vi "maintenancePIP.vi"(8 "error in (no error)":errorcluster) -> (0 "error out":errorcluster, 3 "MAINTENANCE MODE-8, 9, 10, 11":string)   [LabVIEW 2018]
uses:
  Global_1259.vi
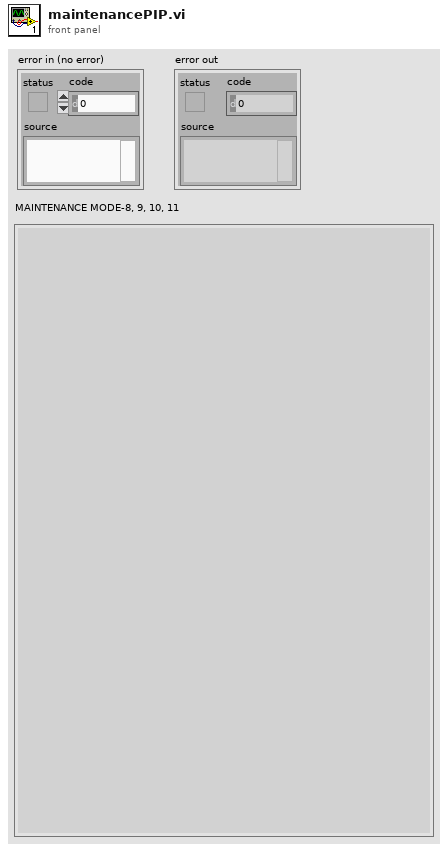
[diagram p1: front panel]
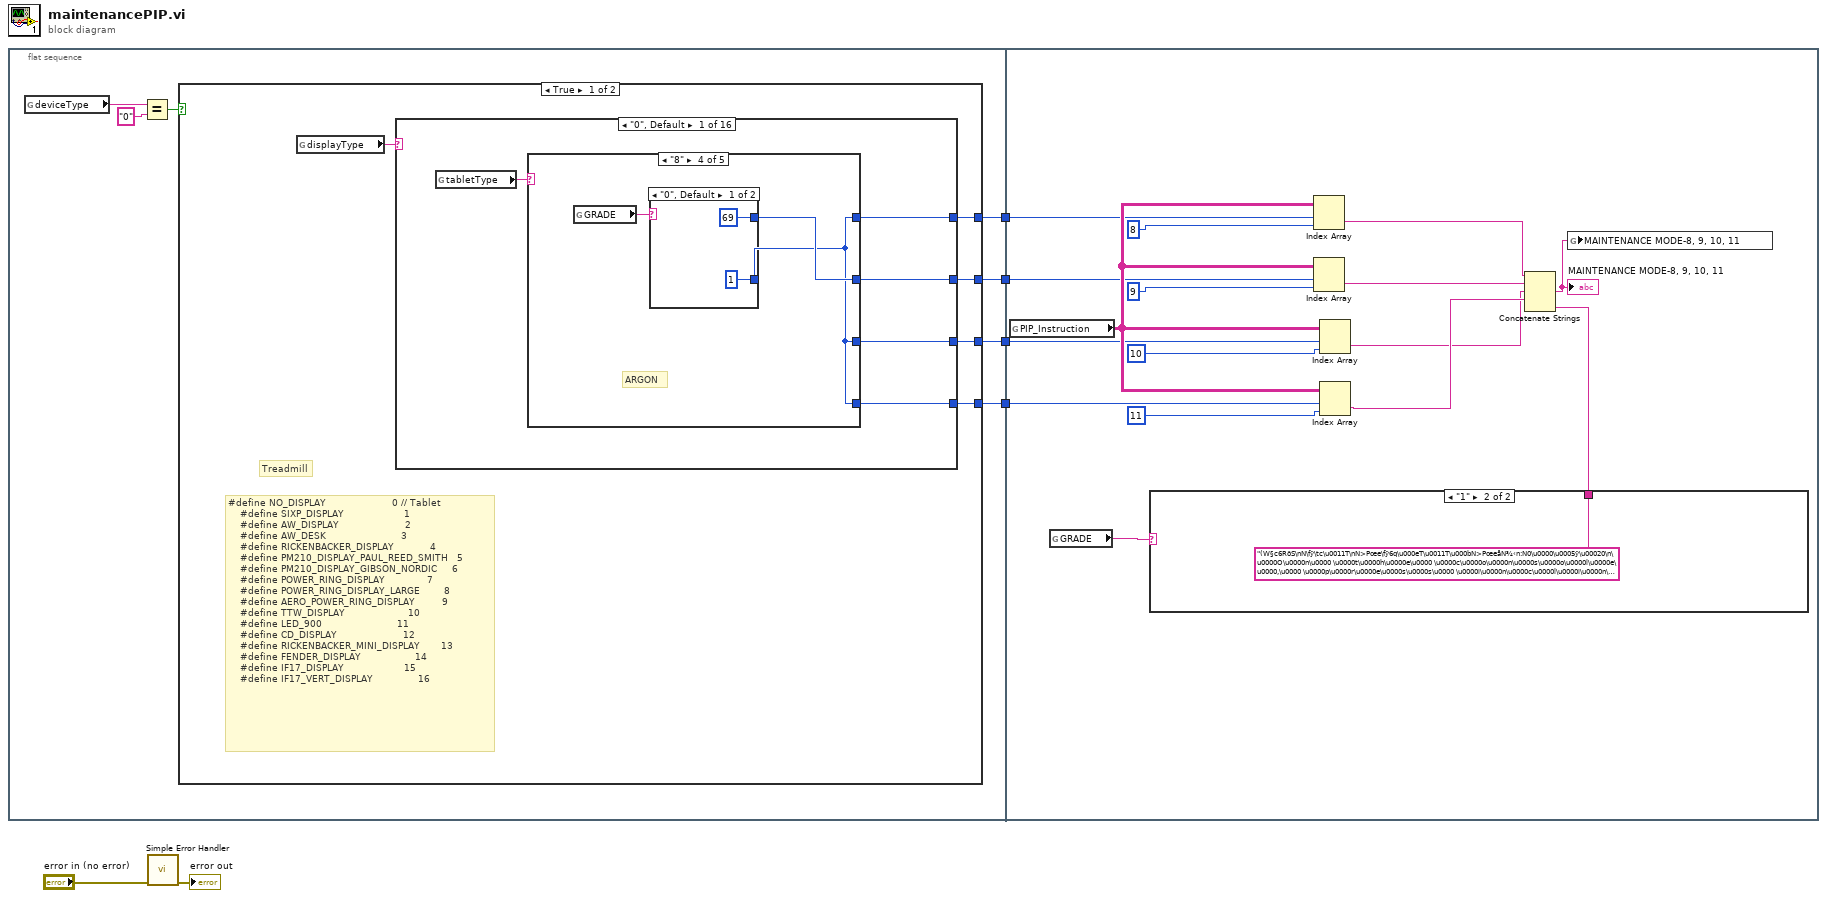
[diagram p0: block diagram]
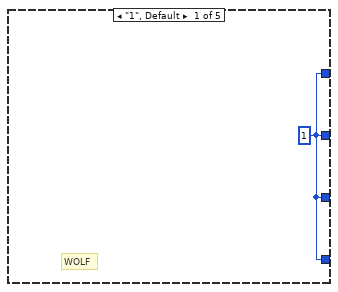
[diagram p2: hidden frame]
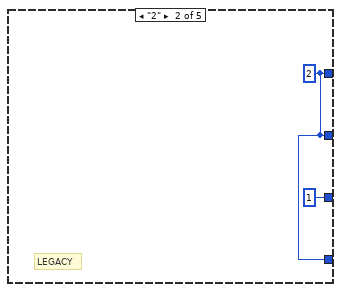
[diagram p3: hidden frame]
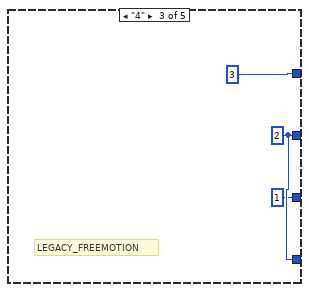
[diagram p4: hidden frame]
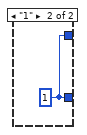
[diagram p5: hidden frame]
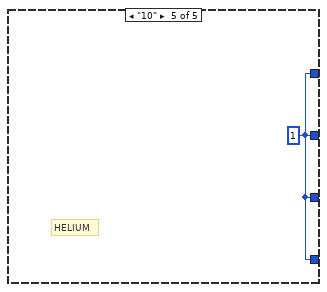
[diagram p6: hidden frame]
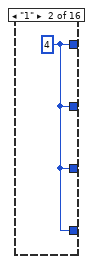
[diagram p7: hidden frame]
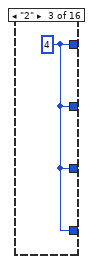
[diagram p8: hidden frame]
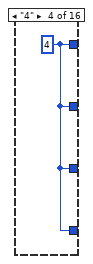
[diagram p9: hidden frame]
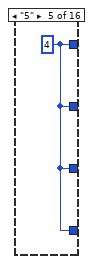
[diagram p10: hidden frame]
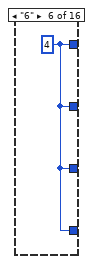
[diagram p11: hidden frame]
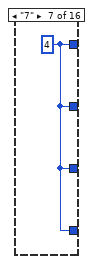
[diagram p12: hidden frame]
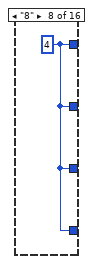
[diagram p13: hidden frame]
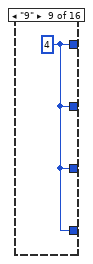
[diagram p14: hidden frame]
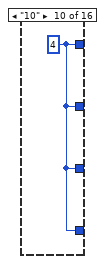
[diagram p15: hidden frame]
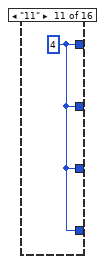
[diagram p16: hidden frame]
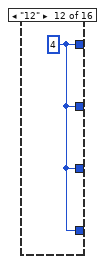
[diagram p17: hidden frame]
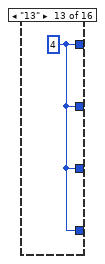
[diagram p18: hidden frame]
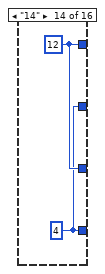
[diagram p19: hidden frame]
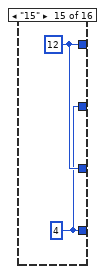
[diagram p20: hidden frame]
diagram:
  n1 = flat-sequence {
    tunnel: [w13] -> w6
    tunnel: [w12] -> w5
    tunnel: [w11] -> w4
    tunnel: [w10] -> w3
    tunnel: w6 -> [w155]
    tunnel: w5 -> [w154]
    tunnel: w4 -> [w153]
    tunnel: w3 -> [w152]
    frame #0 {
      n2 = global read "Global_1259.vi" "deviceType"() -> (w9:string)
      n3 = Equal?(x=w9, y="0") -> (x = y?=w7:bool)
      n4 = case shown="True" w7 {
        tunnel: [w18 w58] -> w13
        tunnel: [w17 w57] -> w12
        tunnel: [w16 w56] -> w11
        tunnel: [w15 w55] -> w10
        frame True {
          # "#define NO_DISPLAY                      0 // Tablet\n    #define SIXP_DISPLAY                    1\n    #define AW_DISPLAY                      2\n    #define AW_DESK                         3\n    #define RICKENBACKER_DISPLAY            4\n    #define PM210_DISPLAY_PAUL_REED_SMITH   5\n    #define PM210_DISPLAY_GIBSON_NORDIC     6\n    #define POWER_RING_DISPLAY              7\n    #define POWER_RING_DISPLAY_LARGE        8\n    #define AERO_POWER_RING_DISPLAY         9\n    #define TTW_DISPLAY                     10\n    #define LED_900                         11\n    #define CD_DISPLAY                      12\n    #define RICKENBACKER_MINI_DISPLAY       13\n    #define FENDER_DISPLAY                  14\n    #define IF17_DISPLAY                    15\n    #define IF17_VERT_DISPLAY               16"
          # "Treadmill"
          n5 = global read "Global_1259.vi" "displayType"() -> (w14:string)
          n6 = case shown="\"0\", Default" w14 {
            tunnel: [w22 w37 w38 w39 w40 w41 w42 w43 w44 w45 w46 w47 w48 w50 w52 w53] -> w18
            tunnel: [w21 w37 w38 w39 w40 w41 w42 w43 w44 w45 w46 w47 w48 w49 w51 w54] -> w17
            tunnel: [w20 w37 w38 w39 w40 w41 w42 w43 w44 w45 w46 w47 w48 w50 w52 w53] -> w16
            tunnel: [w19 w37 w38 w39 w40 w41 w42 w43 w44 w45 w46 w47 w48 w49 w51 w54] -> w15
            frame "0", Default {
              n7 = global read "Global_1259.vi" "tabletType"() -> (w23:string)
              n8 = case shown="\"8\"" w23 {
                tunnel: [w24 w25 w28 w31 w36] -> w21
                tunnel: [w24 w25 3 w30 w36] -> w22
                tunnel: [w24 1 1 w30 w36] -> w20
                tunnel: [w24 w25 w28 w30 w36] -> w19
                frame "1", Default {
                  w24 = 1
                  # "WOLF"
                }
                frame "2" {
                  w25 = 2
                  # "LEGACY"
                }
                frame "4" {
                  w28 = 2
                  # "LEGACY_FREEMOTION"
                }
                frame "8" {
                  # "ARGON"
                  n9 = global read "Global_1259.vi" "GRADE"() -> (w32:string)
                  n10 = case shown="\"0\", Default" w32 {
                    tunnel: [1 w35] -> w30
                    tunnel: [69 w35] -> w31
                    frame "0", Default {
                    }
                    frame "1" {
                      w35 = 1
                    }
                  }
                }
                frame "10" {
                  w36 = 1
                  # "HELIUM"
                }
              }
            }
            frame "1" {
              w37 = 4
            }
            frame "2" {
              w38 = 4
            }
            frame "4" {
              w39 = 4
            }
            frame "5" {
              w40 = 4
            }
            frame "6" {
              w41 = 4
            }
            frame "7" {
              w42 = 4
            }
            frame "8" {
              w43 = 4
            }
            frame "9" {
              w44 = 4
            }
            frame "10" {
              w45 = 4
            }
            frame "11" {
              w46 = 4
            }
            frame "12" {
              w47 = 4
            }
            frame "13" {
              w48 = 4
            }
            frame "14" {
              w49 = 4
              w50 = 12
            }
            frame "15" {
              w51 = 4
              w52 = 12
            }
            frame "16" {
              w54 = 4
              w53 = 12
            }
          }
        }
        frame False {
          # "not treadmill"
          n11 = global read "Global_1259.vi" "displayType"() -> (w61:string)
          n12 = Equal?(x=w61, y="0") -> (x = y?=w59:bool)
          n13 = case shown="False" w59 {
            tunnel: [w65 w123] -> w58
            tunnel: [w66 w122] -> w57
            tunnel: [w64 w121] -> w56
            tunnel: [w63 w120] -> w55
            frame False {
              n14 = global read "Global_1259.vi" "GRADE"() -> (w62:string)
              n15 = case shown="\"0\", Default" w62 {
                tunnel: [w69 w97] -> w66
                tunnel: [w70 w96] -> w65
                tunnel: [w68 w95] -> w64
                tunnel: [w67 w94] -> w63
                frame "0", Default {
                  n16 = global read "Global_1259.vi" "buttonType"() -> (w71:string)
                  n17 = case shown="\"2\"" w71 {
                    tunnel: [8 7 10 7 7 w92] -> w68
                    tunnel: [7 7 10 7 7 w92] -> w67
                    tunnel: [69 69 69 69 69 w92] -> w69
                    tunnel: [8 7 10 8 7 w92] -> w70
                    frame "1", Default {
                    }
                    frame "2" {
                    }
                    frame "4" {
                    }
                    frame "9" {
                    }
                    frame "10" {
                    }
                    frame "12" {
                      w92 = 69
                    }
                  }
                }
                frame "1" {
                  n18 = global read "Global_1259.vi" "buttonType"() -> (w93:string)
                  n19 = case shown="\"2\"" w93 {
                    tunnel: [8 7 10 7 7 w118] -> w95
                    tunnel: [7 7 10 7 7 w118] -> w94
                    tunnel: [7 7 69 8 7 w118] -> w97
                    tunnel: [8 7 10 8 7 w118] -> w96
                    frame "1", Default {
                    }
                    frame "2" {
                    }
                    frame "4" {
                    }
                    frame "9" {
                    }
                    frame "10" {
                    }
                    frame "12" {
                      w118 = 69
                    }
                  }
                }
              }
            }
            frame True {
              n20 = global read "Global_1259.vi" "TABLET"() -> (w119:string)
              n21 = case shown="\"1\", Default" w119 {
                tunnel: [w131 w133 w138 w139 w145] -> w123
                tunnel: [w131 w132 w138 w140 w145] -> w122
                tunnel: [w131 w132 w138 w139 w145] -> w121
                tunnel: [w131 w132 w138 w139 w145] -> w120
                frame "1", Default {
                  w131 = 1
                  n22 = global read "Global_1259.vi" "PIP_Instruction"() -> (w130:string[][])
                  n23 = Index Array(array=w130, index (row)=1 ("disabled index (row)"), index (col)=16 ("disabled index (col)")) -> (element=w129:string)
                  n24 = Index Array(array=w130, index (row)=1 ("disabled index (row)"), index (col)=20 ("disabled index (col)")) -> (element=w128:string)
                  n25 = global write "Global_1259.vi" "USB-16"(w129) -> ()
                  n26 = global write "Global_1259.vi" "TV-20"(w128) -> ()
                }
                frame "2" {
                  n27 = global read "Global_1259.vi" "GRADE"() -> (w134:string)
                  n28 = case shown="\"0\", Default" w134 {
                    tunnel: [1 w137] -> w133
                    tunnel: [69 w137] -> w132
                    frame "0", Default {
                    }
                    frame "1" {
                      w137 = 1
                    }
                  }
                }
                frame "4" {
                  w138 = 1
                }
                frame "8" {
                  n29 = global read "Global_1259.vi" "GRADE"() -> (w141:string)
                  n30 = case shown="\"0\", Default" w141 {
                    tunnel: [1 w144] -> w139
                    tunnel: [69 w144] -> w140
                    frame "0", Default {
                    }
                    frame "1" {
                      w144 = 1
                    }
                  }
                }
                frame "16" {
                  w145 = 1
                }
              }
            }
          }
        }
      }
    }
    frame #1 {
      n31 = global read "Global_1259.vi" "PIP_Instruction"() -> (w161:string[][])
      n32 = global read "Global_1259.vi" "GRADE"() -> (w146:string)
      n33 = case shown="\"1\"" w146 {
        tunnel: ["None" "(W§c6RðS\nN\fÿ\tc\u0011T\nN>Pœe\fÿ6q\u000eT\u0011T\u000bN>PœeåN¾‹n:N0\u0000\u0005ÿ\u00020\n\u0000O\u0000n\u0000 \u0000t\u0000h\u0000e\u0000 \u0000c\u0000o\u0000n\u0000s\u0000o\u0000l\u0000e\u0000,\u0000 \u0000p\u0000r\u0000e\u0000s\u0000s\u0000 \u0000i\u0000n\u0000c\u0000l\u0000i\u0000n\u0000e\u0000 \u0000u\u0000p\u0000 \u0000a\u0000n\u0000d\u0000 \u0000t\u0000h\u0000e\u0000n\u0000 \u0000i\u0000n\u0000c\u0000l\u0000i\u0000n\u0000e\u0000 \u0000d\u0000o\u0000w\u0000n\u0000 \u0000t\u0000o\u0000 \u0000s\u0000e\u0000t\u0000 \u0000t\u0000o\u0000 \u00000\u0000%\u0000.\u0000"] -> w147
        frame "0", Default {
        }
        frame "1" {
        }
      }
      n34 = Index Array(array=w161, index (row)=w155, index (col)=8 ("disabled index (col)")) -> (element=w151:string)
      n35 = Index Array(array=w161, index (row)=w154, index (col)=9 ("disabled index (col)")) -> (element=w150:string)
      n36 = Index Array(array=w161, index (row)=w153, index (col)=10 ("disabled index (col)")) -> (element=w148:string)
      n37 = Index Array(array=w161, index (row)=w152, index (col)=11 ("disabled index (col)")) -> (element=w149:string)
      n38 = Concatenate Strings(w151, w150, w148, w149, w147) -> (w160:string)
      "MAINTENANCE MODE-8, 9, 10, 11" <- w160
      n39 = global write "Global_1259.vi" "MAINTENANCE MODE-8, 9, 10, 11"(w160) -> ()
    }
  }
  n40 = call <vilib>:"Simple Error Handler.vi"("error in (no error)"="error in (no error)") -> ("error out"=→"error out":errorcluster)  [unwired: 4 in, 4 out]
